vi "Connect.vi"(8 "error in (no error)":errorcluster, 11 "Camera Controls in":T1={"Exposure Time (ms)"=27, "cam0 Session"="cam0", "Camera ROI"={"Width"=0, "Height"=0, "Offset X"=0, "Offset Y"=0}, "Command"=""} {"Camera ROI"."Offset Y" max=2046 step=2; "Camera ROI"."Offset X" max=2044 step=4; "Camera ROI"."Height" min=2 max=2048 step=2; "Camera ROI"."Width" min=4 max=2048 step=4; "Exposure Time (ms)" min=27 max=500 step=1 scale=27.0..500.0}) -> (0 "error out":errorcluster, 1 "String":string, 2 "Camera Connected":bool, 3 "Camera Controls out":T1 {"Camera ROI"."Offset Y" max=2046 step=2; "Camera ROI"."Offset X" max=2044 step=4; "Camera ROI"."Height" min=2 max=2048 step=2; "Camera ROI"."Width" min=4 max=2048 step=4; "Exposure Time (ms)" min=27 max=500 step=1 scale=27.0..500.0})   [LabVIEW 2020]
uses:
  _controls/xiCam.ctl
  <vilib>/userDefined/High Color/IMAQdx.ctl
  <vilib>/vision/driver/IMAQdx.llb/IMAQdx Camera Control Mode.ctl
  <vilib>/vision/driver/NI_Vision_Acquisition_Software.lvlib
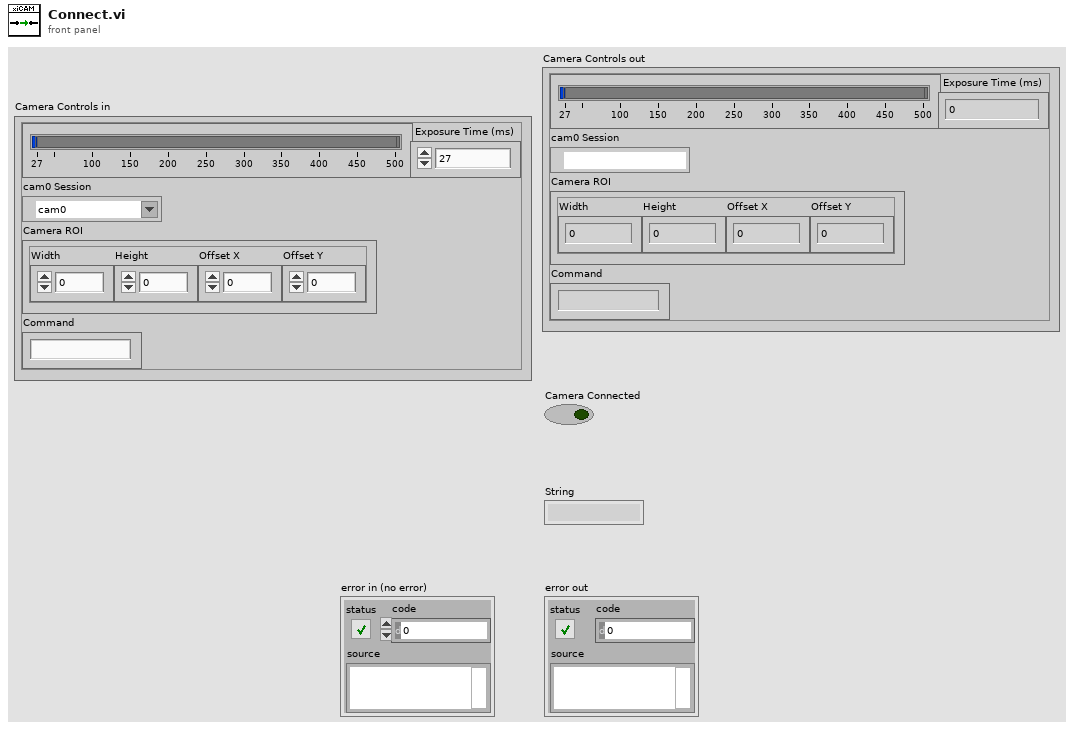
[diagram p1: front panel]
types:
  T1 = typedef "xiCam.ctl" = cluster{"Exposure Time (ms)":u32, "cam0 Session":T2, "Camera ROI":cluster{"Width":u32, "Height":u32, "Offset X":u32, "Offset Y":u32}, "Command":string}
  T2 = typedef "IMAQdx.ctl" = refnum<k21>
  T3 = typedef "NI_Vision_Acquisition_Software.lvlib/IMAQdx Camera Control Mode.ctl" = enum32{"Controller", "Listener"}
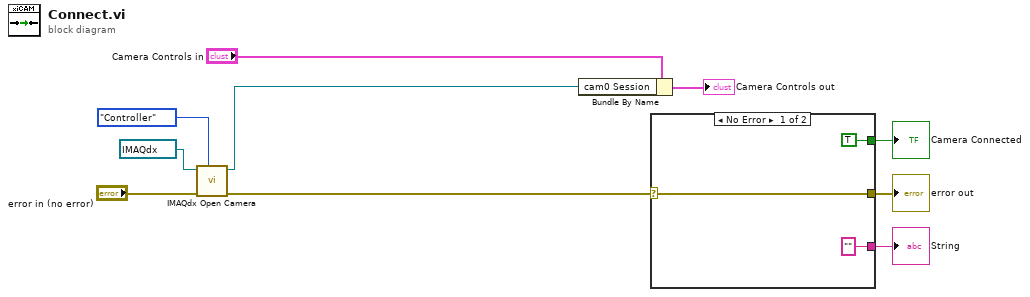
[diagram p0: block diagram]
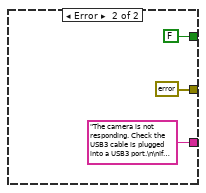
[diagram p2: hidden frame]
diagram:
  n1 = call <vilib>:"IMAQdx Open Camera.vi"("Camera Control Mode"=IMAQdx_Camera_Control_Mode."Controller", "error in"="error in (no error)", "Session In"=T2 "cam0") -> ("error out"=w1:errorcluster, "Session Out"=w2:T2)  [unwired: 7 in]
  n2 = Bundle By Name(cluster="Camera Controls in", "cam0 Session"=w2) -> (→"Camera Controls out":T1)
  n3 = case shown="No Error" w1 {
    selector: w1 -> [w13 _]
    tunnel: [w13 errorcluster {"status"=TRUE, "code"=0, "source"=""} ("error constant")] -> w8
    tunnel: ["" "The camera is not responding. Check the USB3 cable is plugged into a USB3 port.\n\nIf the problem persists contact Arran."] -> w9
    tunnel: [TRUE FALSE] -> w10
    frame No Error {
    }
    frame Error {
    }
  }
  "Camera Connected" <- w10
  "String" <- w9
  "error out" <- w8
